vi "Read Msg Payload.vi"(8 "error in (no error)":errorcluster, 11 "Launch Client Handler Actor Msg in":refnum<class "Launch Client Handler Actor Msg.lvclass">) -> (0 "error out":errorcluster, 1 "timeout ms (5000)":i32, 2 "Remote Address":string, 3 "WebSocket Connection in":refnum<k5>)   [LabVIEW 2016, in "Stream Mediator.lvlib" / "Launch Client Handler Actor Msg.lvclass"]
doc: "--\nCopyright © 2017 Composed SystemsI All rights reserved.\n\nAuthor: Jon McBee <jon.mcbee@composed.io>\n\nThis library is provided \"AS IS\" ,WITHOUT WARRANTIES OR\nCONDITIONS OF ANY KIND, either express or implied.\n\nComposed Systems -- composed.io\n\nStream 0.0.1.1\nJon McBee - Composed Systems\nCopyright (c) 2017, Composed Systems"
uses:
  <userlib>/Composed Systems/Stream/Mediator/Classes/Websocket Server Actor/Websocket Server Msgs/Launch Client Handler Actor Msg/Launch Client Handler Actor Msg.lvclass
  <userlib>/Composed Systems/Stream/Mediator/Classes/Websocket Server Actor/Websocket Server Msgs/Launch Client Handler Actor Msg/Launch Client Handler Actor Msg.lvclass/Launch Client Handler Actor Msg.ctl
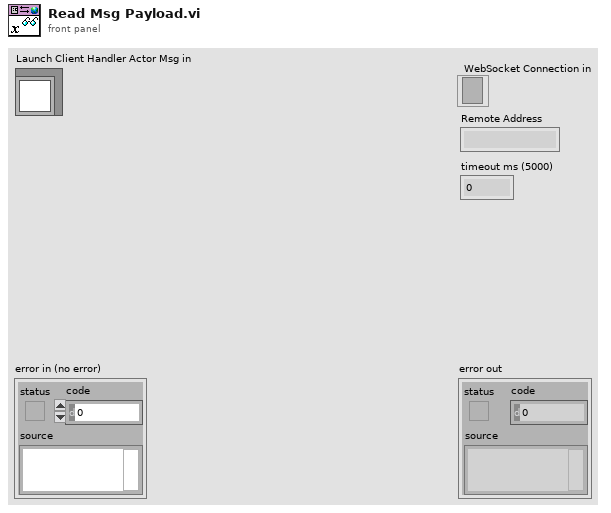
[diagram p1: front panel]
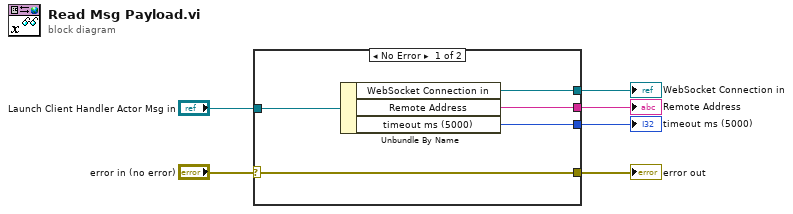
[diagram p0: block diagram]
diagram:
  n1 = case shown="No Error" "error in (no error)" {
    selector: "error in (no error)" -> [w11 w12]
    tunnel: [w11 w12] -> w5
    tunnel: "Launch Client Handler Actor Msg in" -> [w10 _]
    tunnel: [w9 _] -> w3
    tunnel: [w8 _] -> w2
    tunnel: [w7 _] -> w1
    frame No Error {
      n2 = Unbundle By Name(w10) -> ("WebSocket Connection in"=w9:refnum<k5>, "Remote Address"=w8:string, "timeout ms (5000)"=w7:i32)
    }
    frame Error {
    }
  }
  "error out" <- w5
  "WebSocket Connection in" <- w3
  "Remote Address" <- w2
  "timeout ms (5000)" <- w1
